vi "Sentinel Bounds and Origin.vi"() -> (2 "Sentinel Origin":T2, 3 "Sentinel Bounds":T1)   [LabVIEW 2020, in "Choose Implementation Dialog.lvlib"]
uses:
  <vilib>/Utility/miscctls.llb/LVPointTypeDef.ctl
  <vilib>/Utility/miscctls.llb/LVRectTypeDef.ctl
  Choose Implementation Dialog.lvlib
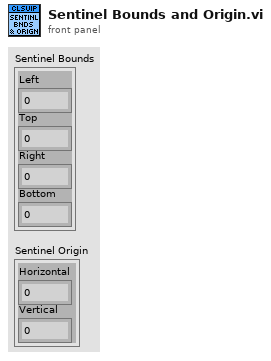
[diagram p1: front panel]
types:
  T1 = typedef "LVRectTypeDef.ctl" = cluster{"Left":i16, "Top":i16, "Right":i16, "Bottom":i16}
  T2 = typedef "LVPointTypeDef.ctl" = cluster{"Horizontal":i16, "Vertical":i16}
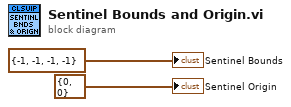
[diagram p0: block diagram]
diagram:
  "Sentinel Origin" <- T2 {"Horizontal"=0, "Vertical"=0} ("Origin out")
  "Sentinel Bounds" <- T1 {"Left"=-1, "Top"=-1, "Right"=-1, "Bottom"=-1} ("Bounds in")
